vi "getFieldValues.vi"(8 "error in (no error)":errorcluster, 11 "IStruct in":refnum<class "IStruct.lvclass">) -> (0 "error out":errorcluster, 2 "Field Values out":refnum<class "IBaseObject.lvclass">[](array[class]), 3 "IStruct out":refnum<class "IStruct.lvclass">)   [LabVIEW 2022 SP3, in "openDAQ.lvlib" / "daqCoreTypes.lvlib" / "IStruct.lvclass"]
uses:
  <instrlib>/openDAQ/Public/Classes/daqCoreTypes/IStruct/IStruct.lvclass
  <instrlib>/openDAQ/Public/Classes/daqCoreTypes/IStruct/IStruct.lvclass/IStruct.ctl
  <instrlib>/openDAQ/Public/Classes/daqCoreTypes/IList/IList.lvclass
  <instrlib>/openDAQ/Public/Classes/daqCoreTypes/IList/Polymorphic/getList/getBaseObjectList.vi
  <instrlib>/openDAQ/Binaries/Windows/x86/copendaq32.dll
  <instrlib>/openDAQ/Public/Classes/IBaseObject/IBaseObject.lvclass
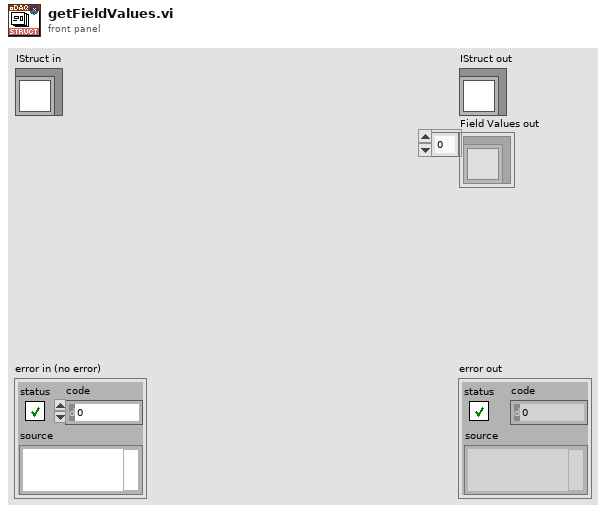
[diagram p1: front panel]
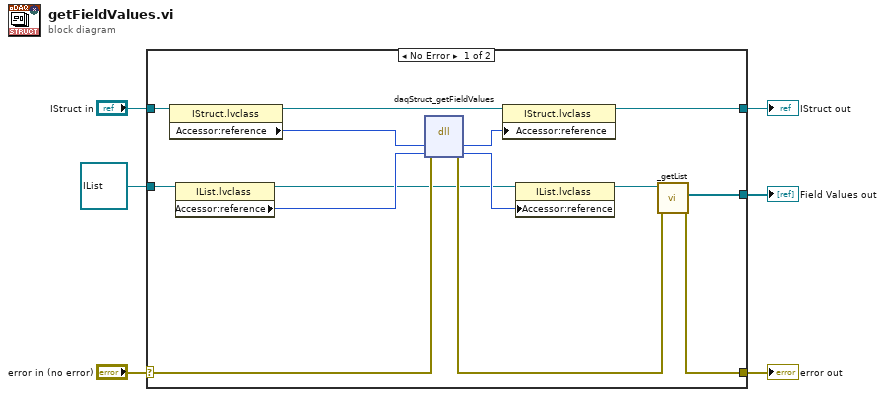
[diagram p0: block diagram]
diagram:
  n1 = case shown="No Error" "error in (no error)" {
    selector: "error in (no error)" -> [w17 w22]
    tunnel: [w8 w22] -> w5
    tunnel: [w13 w21] -> w3
    tunnel: "IStruct in" -> [w16 w21]
    tunnel: refnum<class "IList.lvclass"> refnum ("openDAQ.lvlib:daqCoreTypes.lvlib:IList.lvclass") -> [w10 _]
    tunnel: [w7 _] -> w1
    frame No Error {
      n2 = property class="IStruct.lvclass"(reference=w16) -> (reference out=w14:refnum<class "IStruct.lvclass">, "Accessor:reference"=w15:i64)  [unwired: 1 in, 1 out]
      n3 = property class="IList.lvclass"(reference=w10) -> (reference out=w12:refnum<class "IList.lvclass">, "Accessor:reference"=w18:i64)  [unwired: 1 in, 1 out]
      n4 = dll-call lib="C:/Program Files (x86)/National Instruments/LabVIEW 2022/instr.lib/openDAQ/Binaries/Windows/x86/copendaq*.*" fn="daqStruct_getFieldValues"(error in=w17, "struct"=w15, "values"=w18) -> (error out=w20:errorcluster, "struct"=w11:i64, "values"=w19:i64)  [unwired: 3 in, 1 out]
      n5 = property class="IStruct.lvclass"(reference=w14, "Accessor:reference"=w11) -> (reference out=w13:refnum<class "IStruct.lvclass">)  [unwired: 1 in, 1 out]
      n6 = property class="IList.lvclass"(reference=w12, "Accessor:reference"=w19) -> (reference out=w9:refnum<class "IList.lvclass">)  [unwired: 1 in, 1 out]
      n7 = call-poly <instrlib>:"_getList.vi"("error in (no error)"=w20, "IList in"=w9) -> ("error out"=w8:errorcluster, "baseObjects out"=w7:refnum<class "IBaseObject.lvclass">[])  [unwired: 8 in]
    }
    frame Error {
    }
  }
  "error out" <- w5
  "IStruct out" <- w3
  "Field Values out" <- w1
